vi "WinCI Uninitialize.vi"(8 "error in (no error)":errorcluster) -> (0 "error out":errorcluster)   [LabVIEW 2020, in "NI_SCC_WinCI.lvlib"]
uses:
  <vilib>/SourceControl/Providers/WinCI/NI_SCC_WinCI.lvlib
  <vilib>/SourceControl/support/SCCSup Message Strings GLBL.vi
panel:
  out "result":i32
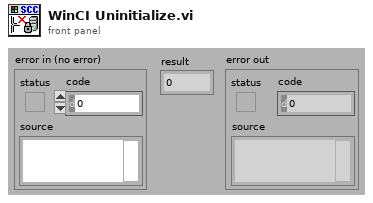
[diagram p1: front panel]
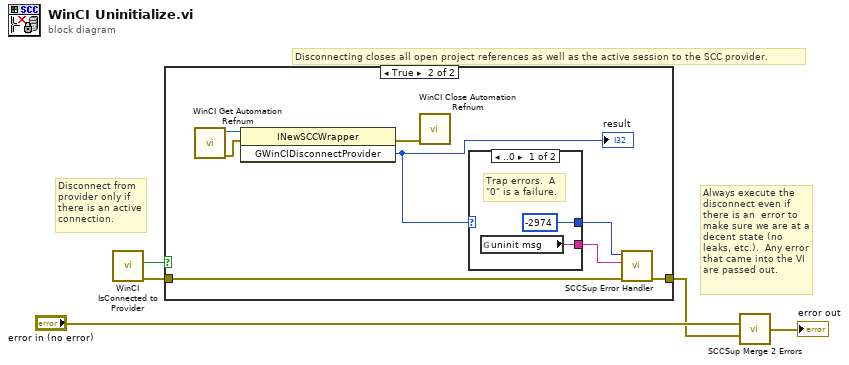
[diagram p0: block diagram]
diagram:
  # "Always execute the disconnect even if there is an  error to make sure we are at a decent state (no leaks, etc.).  Any error that came into the VI are passed out."
  # "Disconnecting closes all open project references as well as the active session to the SCC provider."
  # "Disconnect from provider only if there is an active connection."
  n1 = call <vilib>:"WinCI IsConnected to Provider.vi"() -> ("error out"=w2:errorcluster, "active connection?"=w1:bool)  [unwired: 1 in, 9 out]
  n2 = case shown="True" w1 {
    tunnel: w2 -> [w6 w13]
    tunnel: [w6 w14] -> w4
    frame False {
    }
    frame True {
      n3 = call <vilib>:"WinCI Get Automation Refnum.vi"() -> ("error out"=w9:errorcluster, "automation refnum"=w8:refnum<k7>)  [unwired: 10 out]
      n4 = invoke class="INewSCCWrapper" method="GWinCIDisconnectProvider"(reference=w8, error in=w9) -> (error out=w7:errorcluster, "GWinCIDisconnectProvider"=w10:i32)  [unwired: 1 in, 1 out]
      "result" <- w10
      n5 = call <vilib>:"WinCI Close Automation Refnum.vi"("error in"=w7) -> ()  [unwired: 1 in, 10 out]
      n6 = case shown="..0" w10 {
        tunnel: [-2974 ("result") _] -> w12
        tunnel: [w15 _] -> w11
        frame ..0 {
          # "Trap errors.  A \"0\" is a failure."
          n7 = global read "SCCSup Message Strings GLBL.vi" "uninit msg"() -> (w15:string)
        }
        frame Default {
          # "Function returns 1 for success so treat this as no error."
        }
      }
      n8 = call <vilib>:"SCCSup Error Handler.vi"("error in (no error)"=w13, "operation message"=w11, "scc error code"=w12) -> ("error out"=w14:errorcluster)  [unwired: 1 in, 7 out]
    }
  }
  n9 = call <vilib>:"SCCSup Merge 2 Errors.vi"("Error IO 1"="error in (no error)", "Error IO 2"=w4) -> ("Error IO out"=→"error out":errorcluster)  [unwired: 13 out]
